vi "BMark_Populate Project Ring.vi"(8 "error in (no error)":errorcluster, 11 "Data Cluster in":T1) -> (0 "error out":errorcluster, 3 "Data Cluster out":T1)   [LabVIEW 2016]
uses:
  <resource>/dialog/BookmarkManager/managers/Default/controls/BMark_UI Data.ctl
  <vilib>/addons/analyzer/_analyzerctrls.llb/VIAnCtl Analysis App Info.ctl
  <resource>/dialog/BookmarkManager/managers/Default/controls/BMark_Bookmark Data.ctl
  <resource>/dialog/BookmarkManager/managers/Default/controls/BMark_VI_Identifier.ctl
  <resource>/dialog/BookmarkManager/managers/Default/globals/BMark_User Visible Strings.vi
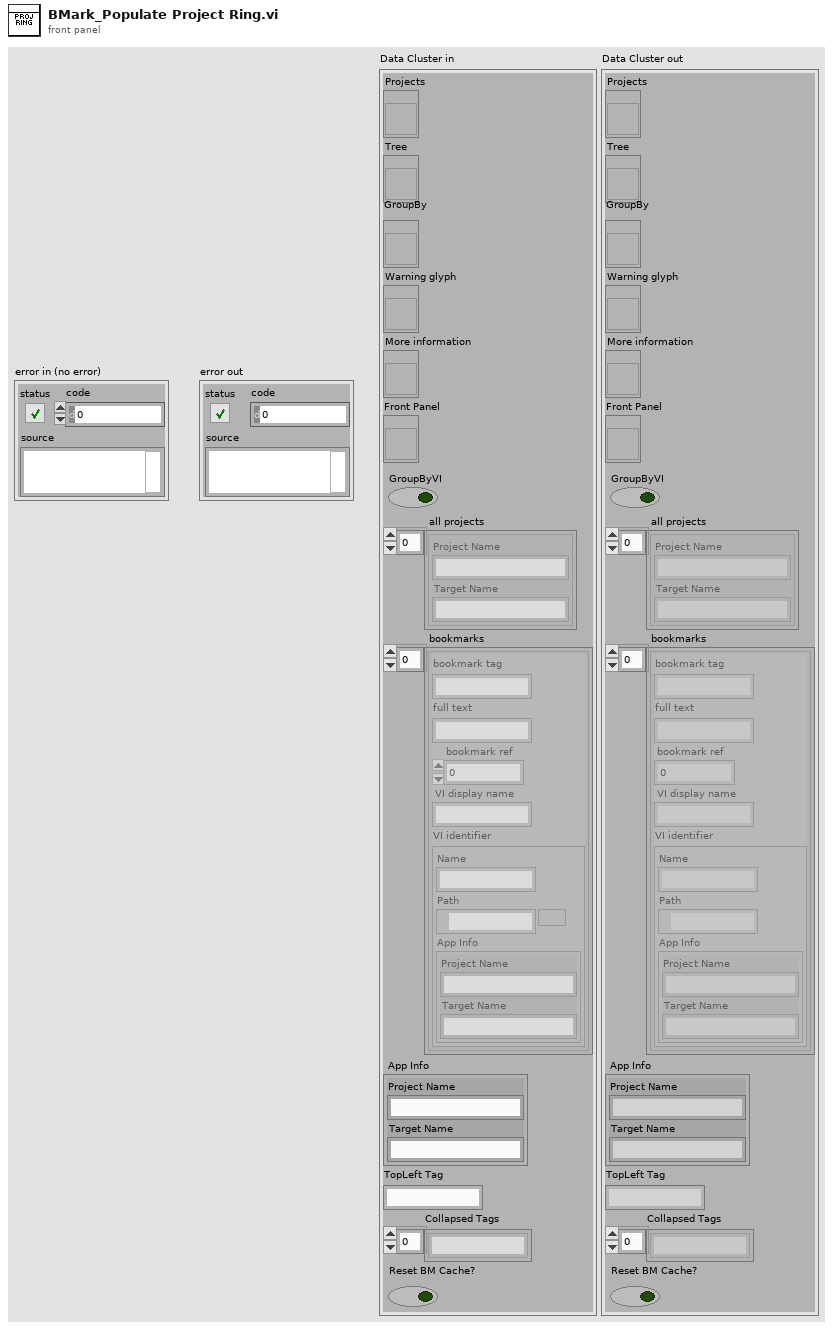
[diagram p1: front panel]
types:
  T1 = typedef "BMark_UI Data.ctl" = cluster{"Projects":refnum<vi>, "Tree":refnum<vi>, "GroupBy":refnum<vi>, "Warning glyph":refnum<vi>, "More information":refnum<vi>, "Front Panel":refnum<vi>, "GroupByVI":bool, "all projects":T2[], "bookmarks":T3[], "App Info":T2, "TopLeft Tag":string, "Collapsed Tags":string[], "Reset BM Cache?":bool}
  T2 = typedef "VIAnCtl Analysis App Info.ctl" = cluster{"Project Name":string, "Target Name":string}
  T3 = typedef "BMark_Bookmark Data.ctl" = cluster{"bookmark tag":string, "full text":string, "bookmark ref":i32, "VI display name":string, "VI identifier":T4}
  T4 = typedef "BMark_VI_Identifier.ctl" = cluster{"Name":string, "Path":path, "App Info":T2}
  T5 = enum8{"Enabled", "Disabled", "Disabled and Grayed Out"}
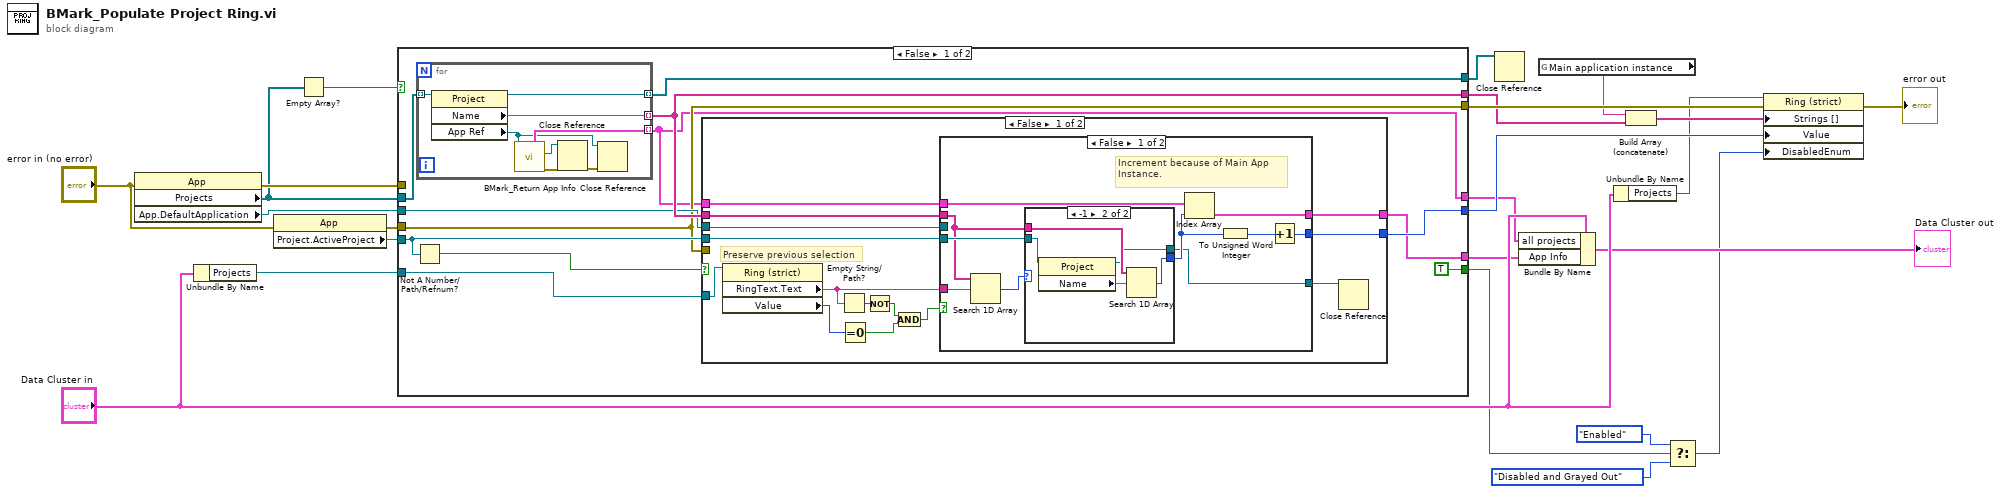
[diagram p0: block diagram]
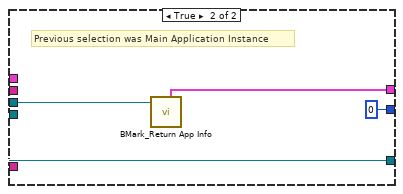
[diagram p3: hidden frame]
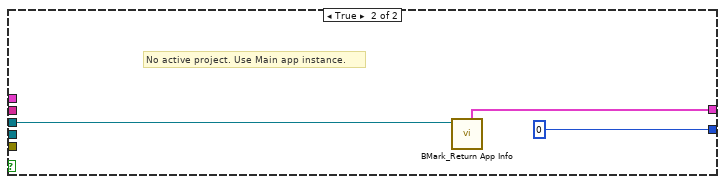
[diagram p4: hidden frame]
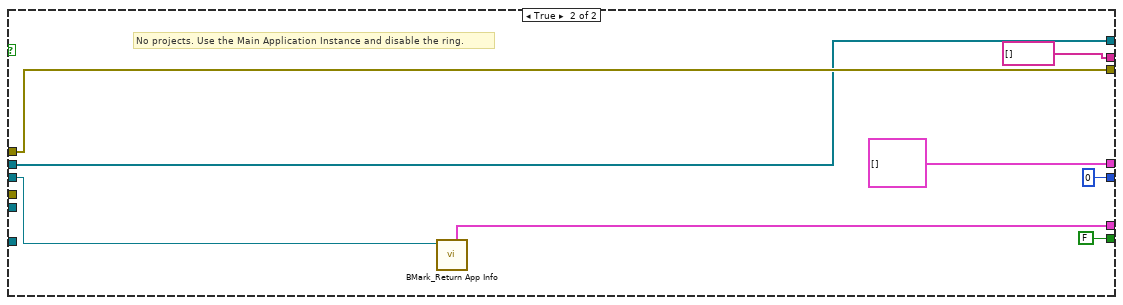
[diagram p5: hidden frame]
diagram:
  n1 = property class="App"(error in="error in (no error)") -> (error out=w15:errorcluster, "Projects"=w14:refnum<vi>[], "App.DefaultApplication"=w16:refnum<vi>)  [unwired: 1 in, 1 out]
  n2 = Unbundle By Name("Data Cluster in") -> ("Projects"=w2:refnum<vi>)
  n3 = property class="App"(error in="error in (no error)") -> (error out=w19:errorcluster, "Project.ActiveProject"=w17:refnum<vi>)  [unwired: 1 in, 1 out]
  n4 = Empty Array?(array=w14) -> (empty?=w13:bool)
  n5 = case shown="False" w13 {
    tunnel: [w29 w90] -> w20
    tunnel: w19 -> [w29 _]
    tunnel: [TRUE FALSE] -> w5
    tunnel: [w33 string[] []] -> w12
    tunnel: [w26 T2[] [] ("all projects")] -> w10
    tunnel: [w32 u16 0] -> w18
    tunnel: w14 -> [w30 w83]
    tunnel: w17 -> [w35 _]
    tunnel: w16 -> [w31 w85]
    tunnel: [w25 w84] -> w9
    tunnel: w15 -> [_ w90]
    tunnel: w2 -> [w28 _]
    tunnel: [w27 w83] -> w1
    frame False {
      n6 = Not A Number/Path/Refnum?(number/path/refnum=w35) -> (NaN/Path/Refnum?=w34:bool)
      n7 = for {
        tunnel: w30 -> [w80] mode=indexing
        tunnel: [w82] -> w33 mode=indexing
        tunnel: [w81] -> w27 mode=indexing
        tunnel: [w79] -> w26 mode=indexing
        n8 = property class="Project"(reference=w80) -> (reference out=w81:refnum<vi>, "Name"=w82:string, "App Ref"=w75:refnum<vi>)  [unwired: 1 in, 1 out]
        n9 = call <resource>:"BMark_Return App Info.vi"("App Refnum in"=w75) -> ("error out"=w78:errorcluster, "App Refnum for Opening VI"=w76:refnum<vi>, "App Info"=w79:T2)  [unwired: 8 in]
        n10 = Close Reference(reference=w76, error in (no error)=w78) -> (error out=w77:errorcluster)
        n11 = Close Reference(reference=w75, error in (no error)=w77) -> ()  [unwired: 1 out]
      }
      n12 = case shown="False" w34 {
        tunnel: w29 -> [_ _]
        tunnel: w33 -> [w46 _]
        tunnel: w35 -> [w47 _]
        tunnel: [w48 u16 0] -> w32
        tunnel: w26 -> [w50 _]
        tunnel: w31 -> [w44 w73]
        tunnel: w28 -> [w49 _]
        tunnel: [w45 w72] -> w25
        frame False {
          # "Preserve previous selection"
          n13 = property class="Ring (strict)"(reference=w49) -> ("RingText.Text"=w40:string, "Value"=w42:u16)  [unwired: 1 in, 2 out]
          n14 = Empty String/Path?(string/path=w40) -> (empty?=w41:bool)
          n15 = Equal To 0?(x=w42) -> (x = 0?=w39:bool)
          n16 = Not(x=w41) -> (.not. x?=w37:bool)
          n17 = And(x=w37, y=w39) -> (x .and. y?=w38:bool)
          n18 = case shown="False" w38 {
            tunnel: w50 -> [w60 _]
            tunnel: w40 -> [w59 _]
            tunnel: [w58 u16 0] -> w48
            tunnel: w47 -> [w55 w68]
            tunnel: w46 -> [w54 _]
            tunnel: [w53 w70] -> w45
            tunnel: w44 -> [_ w71]
            tunnel: [w52 w68] -> w43
            frame False {
              # "Increment because of Main App Instance."
              n19 = Search 1D Array(1D array=w54, element=w59) -> (index of element=w51:i32)  [unwired: 1 in]
              n20 = case shown="-1" w51 {
                selector: w51 -> [w61 _]
                tunnel: [w61 w65] -> w56
                tunnel: w55 -> [w62 w67]
                tunnel: w54 -> [_ w64]
                tunnel: [w62 w63] -> w52
                frame Default {
                }
                frame -1 {
                  n21 = property class="Project"(reference=w67) -> (reference out=w63:refnum<vi>, "Name"=w66:string)  [unwired: 1 in, 1 out]
                  n22 = Search 1D Array(1D array=w64, element=w66) -> (index of element=w65:i32)  [unwired: 1 in]
                }
              }
              n23 = Index Array(array=w60, index=w56) -> (element=w53:T2)
              n24 = To Unsigned Word Integer(number=w56) -> (unsigned 16bit integer=w57:u16)
              n25 = Increment(x=w57) -> (x+1=w58:u16)
            }
            frame True {
              # "Previous selection was Main Application Instance"
              n26 = call <resource>:"BMark_Return App Info.vi"("App Refnum in"=w71) -> ("App Info"=w70:T2)  [unwired: 8 in, 2 out]
            }
          }
          n27 = Close Reference(reference=w43) -> ()  [unwired: 1 in, 1 out]
        }
        frame True {
          # "No active project. Use Main app instance."
          n28 = call <resource>:"BMark_Return App Info.vi"("App Refnum in"=w73) -> ("App Info"=w72:T2)  [unwired: 8 in, 2 out]
        }
      }
    }
    frame True {
      # "No projects. Use the Main Application Instance and disable the ring."
      n29 = call <resource>:"BMark_Return App Info.vi"("App Refnum in"=w85) -> ("App Info"=w84:T2)  [unwired: 8 in, 2 out]
    }
  }
  n30 = Close Reference(reference=w1) -> ()  [unwired: 1 in, 1 out]
  n31 = Bundle By Name(cluster="Data Cluster in", "all projects"=w10, "App Info"=w9) -> (→"Data Cluster out":T1)
  n32 = global read "BMark_User Visible Strings.vi" "Main application instance"() -> (w7:string)
  n33 = Unbundle By Name("Data Cluster in") -> ("Projects"=w8:refnum<vi>)
  n34 = Build Array (concatenate)(w7, w12) -> (w11:string[])
  n35 = Select(t=T5."Enabled" ("Disabled"), s=w5, f=T5."Disabled and Grayed Out" ("Disabled")) -> (s? t:f=w3:T5)
  n36 = property on="Property Node" class="Ring (strict)"(reference=w8, error in=w20, "Strings []"=w11, "Value"=w18, "DisabledEnum"=w3) -> (error out=→"error out":errorcluster)  [unwired: 1 out]
